vi "Fix Window Title.vi"(5 "Project":refnum<vi>, 7 "Project Path":path, 8 "error in":errorcluster, 9 "Path":path=path "../Application Launcher/Splash Screen.vi", 10 "Front Panel Window:Title":string, 11 "Application":refnum<vi>) -> (0 "error out":errorcluster, 3 "dup Application":refnum<vi>)   [LabVIEW 2013, in "TagBusProcessingPluginFeatureDecider.lvclass"]
uses:
  TagBusProcessingPluginFeatureDecider.lvclass
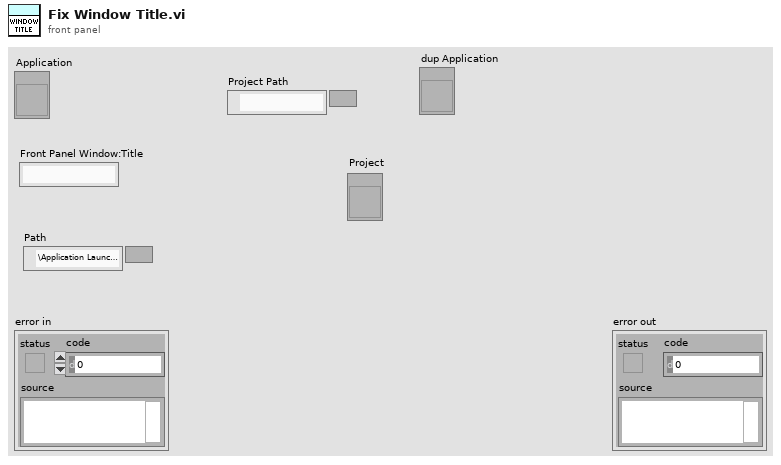
[diagram p1: front panel]
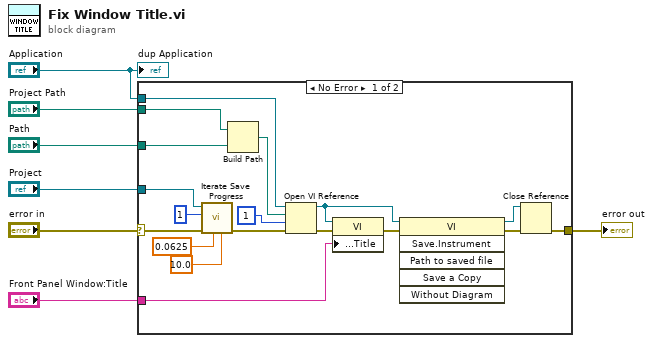
[diagram p0: block diagram]
diagram:
  n1 = case shown="No Error" "error in" {
    selector: "error in" -> [w9 w26]
    tunnel: [w25 w26] -> w7
    tunnel: "Application" -> [w24 _]
    tunnel: "Project Path" -> [w22 _]
    tunnel: "Path" -> [w21 _]
    tunnel: "Front Panel Window:Title" -> [w15 _]
    tunnel: "Project" -> [w8 _]
    frame No Error {
      n2 = call <resource>:"Iterate Save Progress.vi"("Total Iteration Progress"=10.0 ("This Task's Percentage"), "This Task's Percentage"=0.0625, "error in (no error)"=w9, "Total Iterations (this task)"=1, "Project"=w8) -> ("error out"=w10:errorcluster)  [unwired: 6 in]
      n3 = Build Path(base path=w22, name or relative path=w21) -> (appended path=w23:path)
      n4 = Open VI Reference(application reference (local)=w24, vi path=w23, options=1, error in (no error)=w10) -> (vi reference=w17:refnum<vi>, error out=w16:errorcluster)  [unwired: 2 in]
      n5 = property class="VI"(reference=w17, error in=w16, "Front Panel.Title"=w15) -> (error out=w14:errorcluster)  [unwired: 1 out]
      n6 = invoke class="VI" method="Save.Instrument"(reference=w17, error in=w14) -> (reference out=w20:refnum<vi>, error out=w19:errorcluster)  [unwired: 4 in, 4 out]
      n7 = Close Reference(reference=w20, error in (no error)=w19) -> (error out=w25:errorcluster)
    }
    frame Error {
    }
  }
  "error out" <- w7
  "dup Application" <- "Application"
